vi "FA_AgentConfig_GetCloudLookupTime.vi"(8 "Error In":errorcluster) -> (0 "Error Out":errorcluster, 2 "CloudLookupTime":u32)   [LabVIEW 2014, in "FA_AgentConfig.lvlib"]
doc: "Returns the number in miliseconds FlockAgent should wait before contacting the CloudConfig web service to check for new configurations."
uses:
  FA_AgentConfig.lvlib
  FA_LocalStore API/source/VI Source/FA_LocalStore.lvlib
  FA_LocalStore API/source/VI Source/FA_LSSpecialTypes.ctl
  FA_NativeTypes API/source/VI Source/FA_NativeTypes.lvlib
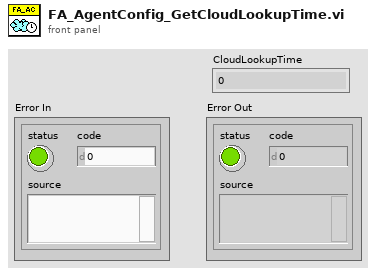
[diagram p1: front panel]
types:
  T1 = typedef "FA_LocalStore.lvlib/FA_LSSpecialTypes.ctl" = string
  T2 = typedef "FA_NativeTypes.lvlib/FA_Config.ctl" = cluster{"Id":string, "Name":T1, "Parameter":cluster{"Name":string, "Value":string}[], "Account":string, "CreateDate":string, "LastModified":string}
  T3 = typedef "FA_AgentConfig.lvlib/FA_AgentConfig.ctl" = cluster{"x-ni-client-id":string, "x-ni-apikey":string, "CloudLookupTime":u32, "Debug":bool, "DeviceName":string}
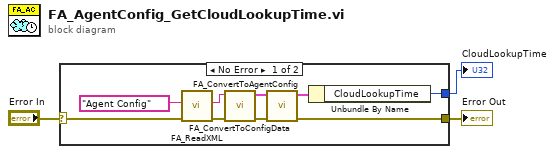
[diagram p0: block diagram]
diagram:
  n1 = case shown="No Error" "Error In" {
    selector: "Error In" -> [w11 w13]
    tunnel: [w9 w13] -> w2
    tunnel: [w10 _] -> w1
    frame No Error {
      n2 = call "FA_ReadXML.vi"("Error In"=w11, "Special Type"=T1 "Agent Config") -> ("Error Out"=w7:errorcluster, "XML String"=w4:string)  [unwired: 6 in]
      n3 = call "FA_ConvertToConfigData.vi"("Error In"=w7, "XML String"=w4) -> ("Error Out"=w6:errorcluster, "ConfigData"=w5:T2)  [unwired: 8 in]
      n4 = call "FA_ConvertToAgentConfig.vi"("Error In"=w6, "Config"=w5) -> ("Error Out"=w9:errorcluster, "AgentConfig"=w8:T3)  [unwired: 8 in]
      n5 = Unbundle By Name(w8) -> ("CloudLookupTime"=w10:u32)
    }
    frame Error {
    }
  }
  "Error Out" <- w2
  "CloudLookupTime" <- w1
